vi "myRIO_BRig_Host_parse_dataTrial__read__v2.vi"(0 "arrayIn_dataTrial":u16[][](array[numeric]), 1 "arrayIn_empty":i32[][](array[numeric])) -> (10 "output_idxUnknown":i32, 11 "output_countTrial":i32, 12 "output_arrayUnknown":i32[][](array[numeric]), 14 "output_idxReward":i32, 15 "output_arrayReward":i32[][](array[numeric]), 16 "output_idxWrong":i32, 17 "output_arrayWrong":i32[][](array[numeric]), 18 "output_idxTimeout":i32, 19 "output_arrayTimeout":i32[][](array[numeric]))   [LabVIEW 2014]
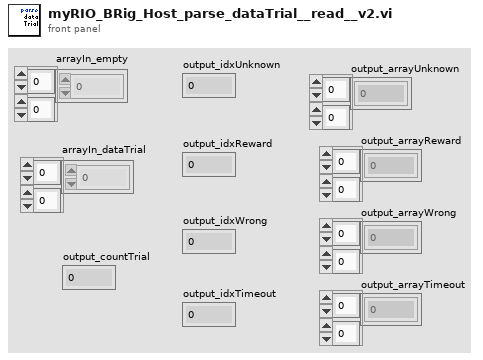
[diagram p1: front panel]
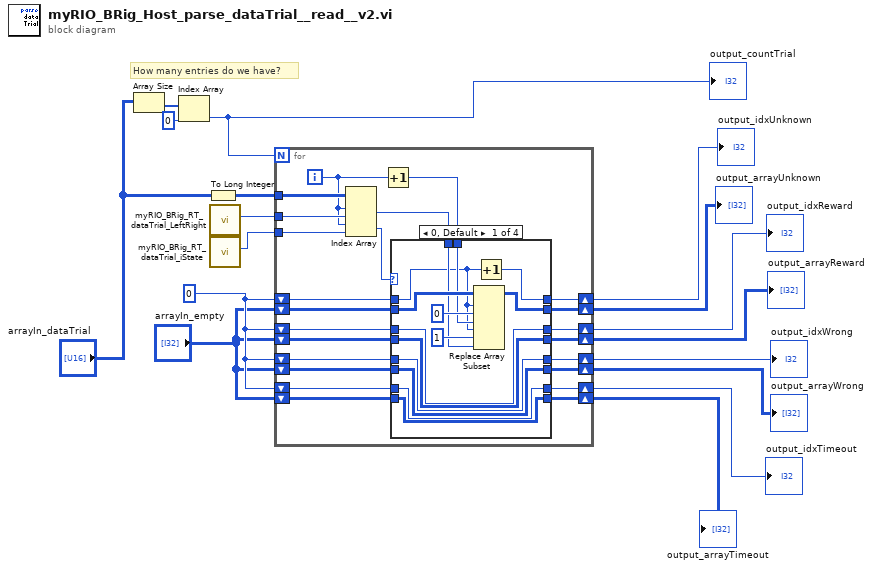
[diagram p0: block diagram]
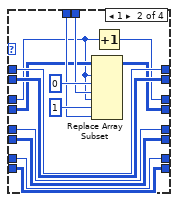
[diagram p2: hidden frame]
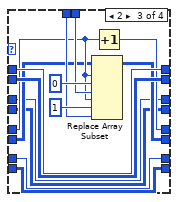
[diagram p3: hidden frame]
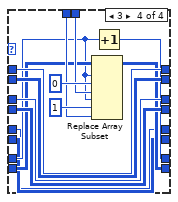
[diagram p4: hidden frame]
diagram:
  w12 = 0
  # "How many entries do we have?"
  n1 = Array Size(array="arrayIn_dataTrial") -> (size(s)=w16:i32[])
  n2 = Index Array(array=w16, index=0) -> (element=w1:i32)
  "output_countTrial" <- w1
  n3 = To Long Integer(number="arrayIn_dataTrial") -> (32bit integer=w13:i32[][])
  n4 = call "myRIO_BRig_RT_dataTrial_LeftRight.vi"() -> ("output_LeftRight"=w15:i32)  [unwired: 11 in]
  n5 = call "myRIO_BRig_RT_dataTrial_iState.vi"() -> ("output_iState"=w14:i32)  [unwired: 11 in]
  n6 = for {
    N: w1 -> [_]
    tunnel: w13 -> [w40]
    tunnel: w15 -> [w39]
    tunnel: w14 -> [w38]
    shift-right: [w31] -> w10
    shift-left: w12 -> [w35]
    shift-right: [w30] -> w9
    shift-left: "arrayIn_empty" -> [w34]
    shift-right: [w18] -> w8
    shift-left: w12 -> [w29]
    shift-right: [w19] -> w7
    shift-left: "arrayIn_empty" -> [w28]
    shift-right: [w20] -> w6
    shift-left: w12 -> [w27]
    shift-right: [w21] -> w5
    shift-left: "arrayIn_empty" -> [w26]
    shift-right: [w22] -> w4
    shift-left: w12 -> [w25]
    shift-right: [w23] -> w3
    shift-left: "arrayIn_empty" -> [w24]
    i -> [w37]
    n7 = Index Array(array=w40, index (row) #1=w37, index (col) #1=w39, index (row) #2=w37, index (col) #2=w38) -> (element #1=w33:i32, element #2=w36:i32)
    n8 = Increment(x=w37) -> (x+1=w32:i32)
    n9 = case shown="0, Default" w36 {
      tunnel: w35 -> [w41 w60 w76 w92]
      tunnel: w34 -> [w54 w59 w75 w91]
      tunnel: w33 -> [w51 w66 w80 w94]
      tunnel: w32 -> [w50 w65 w79 w93]
      tunnel: [w49 w60 w76 w92] -> w31
      tunnel: [w48 w59 w75 w91] -> w30
      tunnel: w29 -> [w42 w57 w70 w90]
      tunnel: w28 -> [w43 w58 w69 w89]
      tunnel: w27 -> [w44 w61 w74 w83]
      tunnel: w26 -> [w45 w62 w73 w84]
      tunnel: w25 -> [w46 w63 w77 w87]
      tunnel: w24 -> [w47 w64 w78 w88]
      tunnel: [w47 w64 w78 w85] -> w23
      tunnel: [w46 w63 w77 w86] -> w22
      tunnel: [w45 w62 w71 w84] -> w21
      tunnel: [w44 w61 w72 w83] -> w20
      tunnel: [w43 w55 w69 w89] -> w19
      tunnel: [w42 w56 w70 w90] -> w18
      frame 0, Default {
        n10 = Replace Array Subset(array=w54, new element #1=w50, index (row) #1=w41, index (col) #1=0 ("disabled index (col)"), new element #2=w51, index (row) #2=w41, index (col) #2=1 ("disabled index (col)")) -> (w48:i32[][])
        n11 = Increment(x=w41) -> (x+1=w49:i32)
      }
      frame 1 {
        n12 = Replace Array Subset(array=w58, new element #1=w65, index (row) #1=w57, index (col) #1=0 ("disabled index (col)"), new element #2=w66, index (row) #2=w57, index (col) #2=1 ("disabled index (col)")) -> (w55:i32[][])
        n13 = Increment(x=w57) -> (x+1=w56:i32)
      }
      frame 2 {
        n14 = Replace Array Subset(array=w73, new element #1=w79, index (row) #1=w74, index (col) #1=0 ("disabled index (col)"), new element #2=w80, index (row) #2=w74, index (col) #2=1 ("disabled index (col)")) -> (w71:i32[][])
        n15 = Increment(x=w74) -> (x+1=w72:i32)
      }
      frame 3 {
        n16 = Replace Array Subset(array=w88, new element #1=w93, index (row) #1=w87, index (col) #1=0 ("disabled index (col)"), new element #2=w94, index (row) #2=w87, index (col) #2=1 ("disabled index (col)")) -> (w85:i32[][])
        n17 = Increment(x=w87) -> (x+1=w86:i32)
      }
    }
  }
  "output_idxUnknown" <- w10
  "output_arrayUnknown" <- w9
  "output_idxReward" <- w8
  "output_arrayReward" <- w7
  "output_idxWrong" <- w6
  "output_arrayWrong" <- w5
  "output_idxTimeout" <- w4
  "output_arrayTimeout" <- w3
